vi "读取-Phone个人客户端集.vi"(8 "error in (no error)":errorcluster caption="错误输入（无错误）", 11 "客户单位输入":refnum<class "客户单位.lvclass">) -> (0 "error out":errorcluster caption="错误输出", 2 "Phone个人客户端集":refnum<class "Phone个人客户端.lvclass">[](array[class]), 3 "客户单位输出":refnum<class "客户单位.lvclass">)   [LabVIEW 2013, in "客户单位.lvclass"]
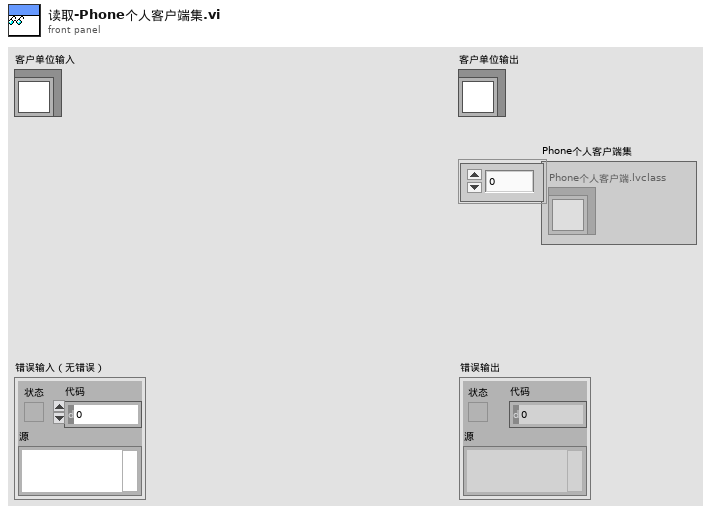
[diagram p1: front panel]
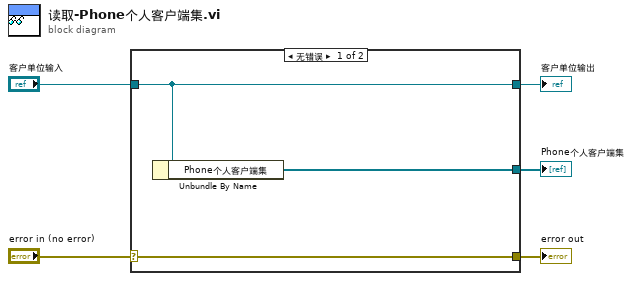
[diagram p0: block diagram]
diagram:
  n1 = case shown="无错误" "error in (no error)" {
    selector: "error in (no error)" -> [w8 w9]
    tunnel: [w8 w9] -> w4
    tunnel: [w7 w10] -> w2
    tunnel: "客户单位输入" -> [w7 w10]
    tunnel: [w6 _] -> w1
    frame No Error {
      n2 = Unbundle By Name(w7) -> ("Phone个人客户端集"=w6:refnum<class "Phone个人客户端.lvclass">[])
    }
    frame Error {
    }
  }
  "error out" <- w4
  "客户单位输出" <- w2
  "Phone个人客户端集" <- w1
